vi "计算三阶正图像.vi"(0 "关联成像原理":dbl, 5 "重建方法":dbl, 7 "光源散斑簇":T1, 9 "差分计算一维矩阵":dbl[](array[numeric]), 11 "正图像筛选门限":dbl) -> (4 "未归一化三阶正图像":dbl[][](array[numeric]))   [LabVIEW 2018]
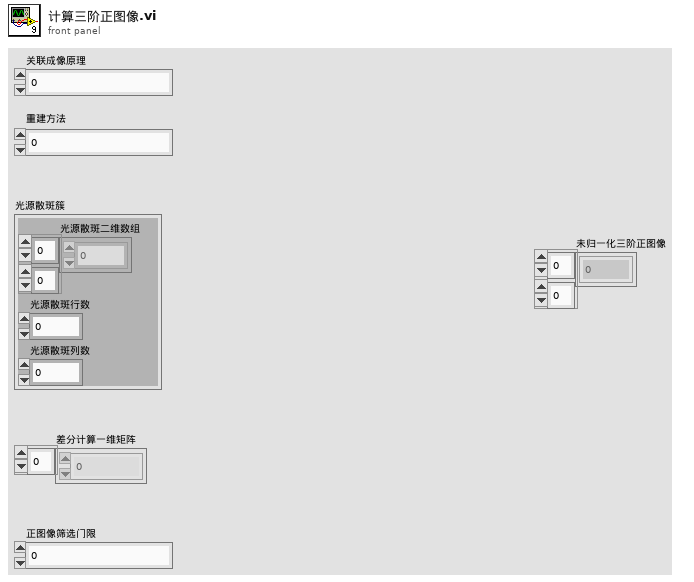
[diagram p1: front panel]
types:
  T1 = cluster{"光源散斑二维数组":dbl[][], "光源散斑行数":i32, "光源散斑列数":i32}
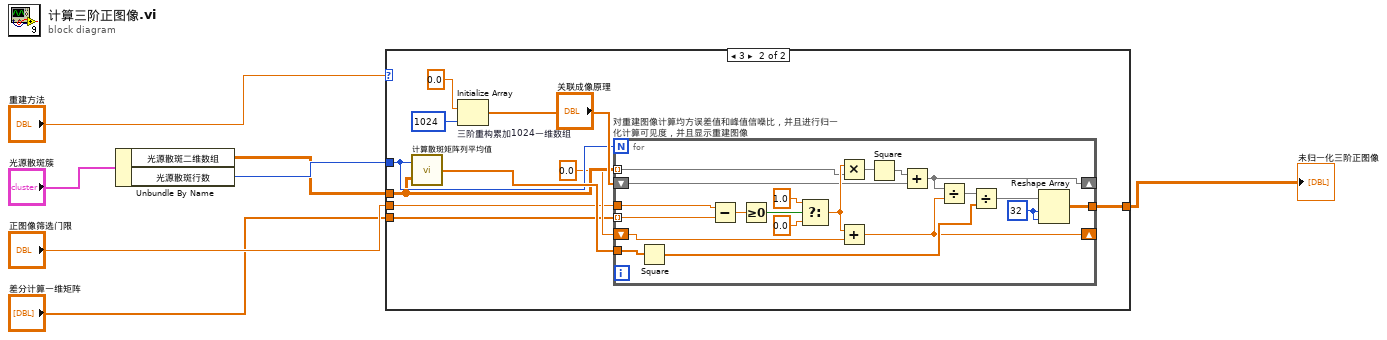
[diagram p0: block diagram]
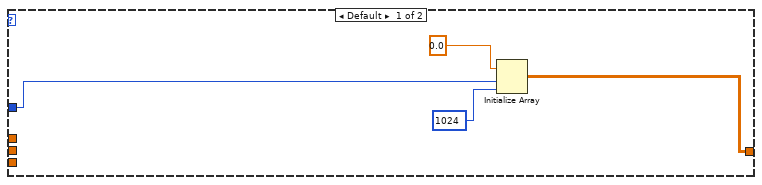
[diagram p2: hidden frame]
diagram:
  n1 = Unbundle By Name("光源散斑簇") -> ("光源散斑二维数组"=w1:dbl[][], "光源散斑行数"=w2:i32)
  n2 = case shown="3" "重建方法" {
    tunnel: w1 -> [_ w16]
    tunnel: w2 -> [w10 w17]
    tunnel: "正图像筛选门限" -> [_ w14]
    tunnel: "差分计算一维矩阵" -> [_ w13]
    tunnel: [w8 w12] -> w4
    frame Default {
      n3 = Initialize Array(0.0, w10, 1024) -> (w8:dbl[][])
    }
    frame 3 {
      n4 = call "计算散斑矩阵列平均值.vi"("散斑二维数组"=w16, "散斑二维数组行数"=w17) -> ("散斑二维数组列平均值"=w21:dbl[])
      n5 = Initialize Array "三阶重构累加1024一维数组"(0.0 ("元素"), 1024 ("维数大小")) -> (w20:dbl[])
      n6 = for "对重建图像计算均方误差值和峰值信噪比，并且进行归一化计算可见度，并且显示重建图像" {
        N: w17 -> [_]
        tunnel: w16 -> [w22] mode=indexing
        shift-right: [w24] -> _
        shift-left: 0.0 ("数值") -> [w35]
        tunnel: w14 -> [w41]
        tunnel: w21 -> [w27]
        shift-right: [w30] -> _
        shift-left: w20 -> [w31]
        tunnel: [w25] -> w12
        tunnel: w13 -> [w23] mode=indexing
        w34 = 32 ("维数大小")
        n7 = Square(x=w27) -> (x^2=w26:dbl[])
        n8 = Subtract(x=w41, y=w23) -> (x-y=w37:dbl)
        n9 = Greater Or Equal To 0?(x=w37) -> (x >= 0?=w40:bool)
        n10 = Select(t=1.0, s=w40, f=0.0) -> (s? t:f=w36:dbl)
        n11 = Multiply(x=w36, y=w22) -> (x*y=w33:dbl[])
        n12 = Add(x=w36, y=w35) -> (x+y=w24:dbl)
        n13 = Square(x=w33) -> (x^2=w32:dbl[])
        n14 = Add(x=w32, y=w31) -> (x+y=w30:dbl[])
        n15 = Divide(x=w30, y=w24) -> (x/y=w29:dbl[])
        n16 = Divide(x=w29, y=w26) -> (x/y=w28:dbl[])
        n17 = Reshape Array(w28, w34, w34) -> (w25:dbl[][])
      }
    }
  }
  "未归一化三阶正图像" <- w4
